vi "HVBuncher.contents.vi"   [LabVIEW 2014, in "HVBuncher.lvlib"]
uses:
  HVBuncher.lvlib
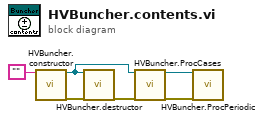
[diagram p0: block diagram]
diagram:
  n1 = call "HVBuncher.constructor.vi"("name"="") -> ("i ref out"=w3:refnum<vi>, "error out"=w6:errorcluster)  [unwired: 16 in, 1 out]
  n2 = call "HVBuncher.destructor.vi"("i ref in"=w3, "error in (no error)"=w6) -> ("error out"=w5:errorcluster)  [unwired: 17 in]
  n3 = call "HVBuncher.ProcCases.vi"("i ref in"=w3, "error in (no error)"=w5) -> ("i ref out"=w2:refnum<vi>, "error out"=w4:errorcluster)  [unwired: 15 in, 1 out]
  n4 = call "HVBuncher.ProcPeriodic.vi"("i ref in"=w2, "error in (no error)"=w4) -> ()  [unwired: 15 in, 3 out]
